vi "Configure Controller.vi"(9 "WindowHandle":i32, 10 "Config File Path":path=path "MeasurementConfig.ini") -> (0 "error IO":errorcluster, 2 "Absolute Path":path, 4 "Canceled?":bool)   [LabVIEW 2016, in "Controller API.lvlib" / "Controller API.lvclass"]
uses:
  <userlib>/Measurement Utility API/Controller API.lvclass
  <userlib>/Common Components/Msmt Configuration/Controller Configuration.lvclass
  C:/Program Files (x86)/National Instruments/LabVIEW 2016/user.lib/Configuration Dialog Actor/Configuration.lvclass
  C:/Program Files (x86)/National Instruments/LabVIEW 2016/vi.lib/ActorFramework/Actor/Actor.lvclass
  <vilib>/ActorFramework/LastAck/Last Ack.lvclass
  <vilib>/ActorFramework/Message Queue/Message Queue.lvclass/Message Queue.ctl
  <vilib>/ActorFramework/Message Dequeuer/Message Dequeuer.lvclass/Message Dequeuer.ctl
  <vilib>/ActorFramework/LastAck/Last Ack.lvclass/Last Ack.ctl
  <userlib>/Configuration Dialog Actor/Configuration.lvclass/Configuration.ctl
  <vilib>/ActorFramework/Message Priority Queue/Priority Dequeue.vi
  <userlib>/Configuration Dialog Actor/Configuration.lvclass
  <vilib>/ActorFramework/Actor/Actor.lvclass
  <vilib>/ActorFramework/Message Queue/Message Queue.lvclass
  <vilib>/ActorFramework/Message Dequeuer/Message Dequeuer.lvclass
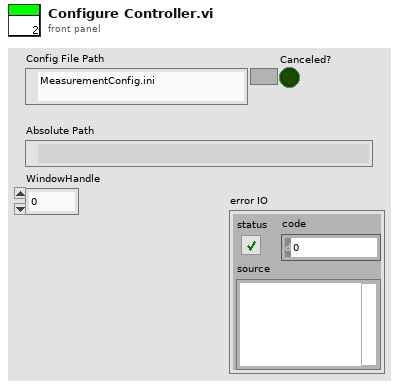
[diagram p1: front panel]
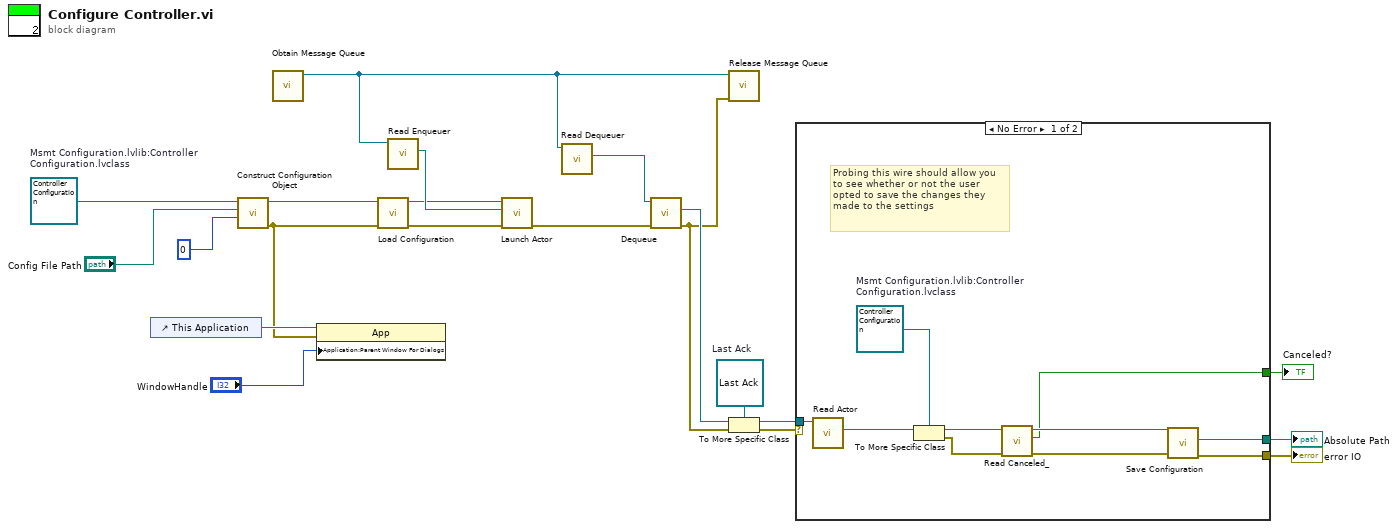
[diagram p0: block diagram]
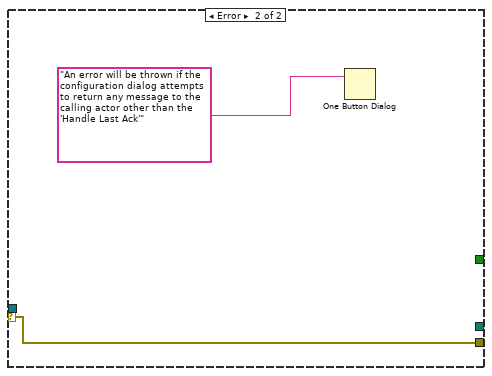
[diagram p2: hidden frame]
diagram:
  w15 = refnum<class "Last Ack.lvclass"> refnum  # Last Ack
  w21 = refnum<class "Controller Configuration.lvclass"> refnum  # Msmt Configuration.lvlib:Controller Configuration.lvclass
  n1 = control-ref of="This Application"() -> (w3:refnum<vi>)
  n2 = call <userlib>:"Construct Configuration Object.vi"("Initial Category Selection"=0, "Configuration File Path"="Config File Path", "Configuration in"=w21) -> ("error out"=w2:errorcluster, "Configuration out"=w19:refnum<class "Controller Configuration.lvclass">)  [unwired: 5 in, 2 out]
  n3 = call <vilib>:"Obtain Message Queue.vi"() -> ("Message Queue"=w17:refnum<class "Message Queue.lvclass">)  [unwired: 10 in, 1 out]
  n4 = property class="App"(reference=w3, error in=w2, "Application:Parent Window For Dialogs"="WindowHandle") -> ()  [unwired: 2 out]
  n5 = call <userlib>:"Load Configuration.vi"("error in (no error)"=w2, "Configuration in"=w19) -> ("error out"=w7:errorcluster, "Configuration out"=w6:refnum<class "Controller Configuration.lvclass">)  [unwired: 7 in, 1 out]
  n6 = call <vilib>:"Read Enqueuer.vi"("Message Queue"=w17) -> ("Message Enqueuer"=w18:refnum<class "Message Enqueuer.lvclass">)  [unwired: 10 in]
  n7 = call <vilib>:"Launch Actor.vi"("error in (no error)"=w7, "Actor-to-Caller Enqueuer"=w18, "Actor"=w6) -> ("error out"=w11:errorcluster)  [unwired: 7 in, 1 out]
  n8 = call <vilib>:"Read Dequeuer.vi"("Message Queue"=w17) -> ("Message Dequeuer"=w12:refnum<class "Message Dequeuer.lvclass">)  [unwired: 10 in]
  n9 = call <vilib>:"Dequeue.vi"("error in (no error)"=w11, "Message Dequeuer in"=w12) -> ("error out"=w10:errorcluster, "Message"=w16:refnum<class "Message.lvclass">)  [unwired: 5 in, 3 out]
  n10 = call <vilib>:"Release Message Queue.vi"("error in (no error)"=w10, "Message Queue"=w17) -> ()  [unwired: 8 in, 2 out]
  n11 = To More Specific Class(target class=w15, reference=w16, error in=w10) -> (specific class reference=w14:refnum<class "Last Ack.lvclass">, error out=w13:errorcluster)
  n12 = case shown="No Error" w13 {
    selector: w13 -> [_ w32]
    tunnel: w14 -> [w31 _]
    tunnel: [w29 w32] -> w9
    tunnel: [w28 _] -> w8
    tunnel: [w22 _] -> w1
    frame No Error {
      w27 = refnum<class "Controller Configuration.lvclass"> refnum  # Msmt Configuration.lvlib:Controller Configuration.lvclass
      # "Probing this wire should allow you to see whether or not the user opted to save the changes they made to the settings"
      n13 = call <vilib>:"Read Actor.vi"("Last Ack"=w31) -> ("Actor"=w30:refnum<class "Actor.lvclass">)  [unwired: 10 in]
      n14 = To More Specific Class(target class=w27, reference=w30) -> (specific class reference=w26:refnum<class "Controller Configuration.lvclass">, error out=w24:errorcluster)  [unwired: 1 in]
      n15 = call <vilib>:"Read Canceled_.vi"("error in (no error)"=w24, "Configuration in"=w26) -> ("error out"=w23:errorcluster, "Canceled?"=w22:bool, "Configuration out"=w25:refnum<class "Controller Configuration.lvclass">)  [unwired: 7 in]
      n16 = call <userlib>:"Save Configuration.vi"("error in (no error)"=w23, "Configuration in"=w25) -> ("error out"=w29:errorcluster, "file path"=w28:path)  [unwired: 7 in, 1 out]
    }
    frame Error {
      n17 = One Button Dialog(message="An error will be thrown if the configuration dialog attempts to return any message to the calling actor other than the 'Handle Last Ack'") -> ()  [unwired: 1 in, 1 out]
    }
  }
  "error IO" <- w9
  "Absolute Path" <- w8
  "Canceled?" <- w1
